vi "DFT.vi"() -> ()   [LabVIEW 2014]
panel:
  out "Magnitude Response":dbl[](graph)
  out "DFT Output X(k)":cdb[](array[numeric])
  out "WN":cdb[](array[numeric])
  in  "Input array x(n)":dbl[](array[numeric])
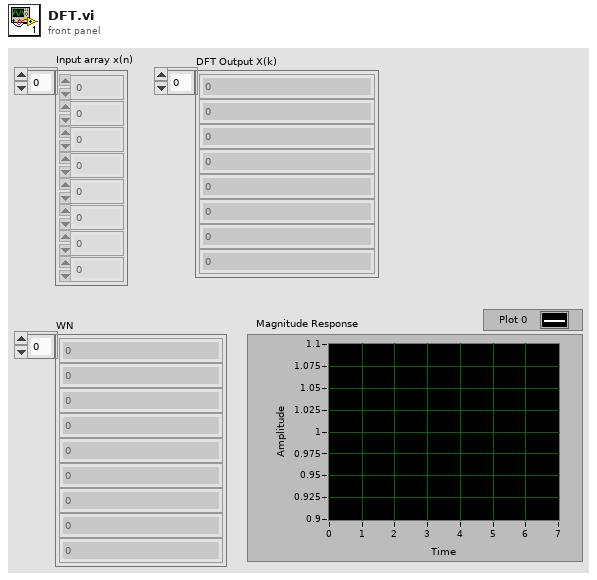
[diagram p1: front panel]
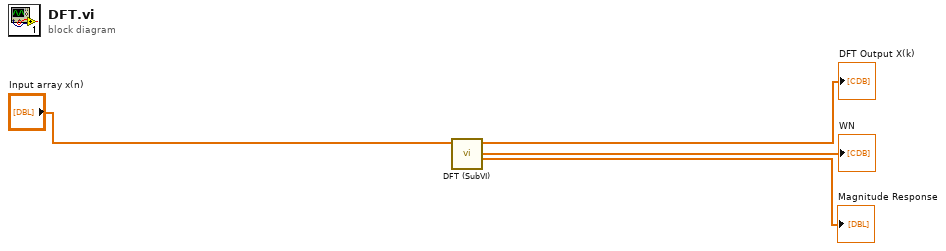
[diagram p0: block diagram]
diagram:
  n1 = call "DFT (SubVI).vi"("Input array x(n)"="Input array x(n)") -> ("Magnitude of X(k)"=→"Magnitude Response":dbl[], "WN"=→"WN":cdb[], "DFT Output X(k)"=→"DFT Output X(k)":cdb[])  [unwired: 8 in]
